vi "Get Config.vi"(8 "error in (no error)":errorcluster, 11 "SimSyA in":refnum<class "SimSyA.lvclass">) -> (0 "error out":errorcluster, 1 "Config Data":variant, 3 "SimSyA out":refnum<class "SimSyA.lvclass">)   [LabVIEW 2014, in "SimSyA.lvlib" / "SimSyA.lvclass"]
uses:
  SimSyA.lvclass
  DriverMasterSync/build/DriverMasterSync.lvlibp/Modules/HAL/DriverMasterSync/DriverMasterSyncClass/DriverMasterSync.lvclass
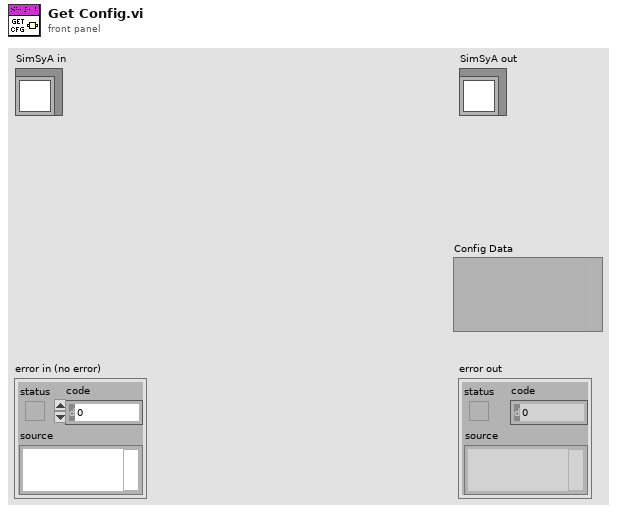
[diagram p1: front panel]
types:
  T1 = typedef "DriverMasterSync.lvlibp/HAL Config Data.ctl" = cluster{"HWSync Index":u32, "Driver Name":string, "Channel Mask":u64}
  T2 = cluster{"Channel Mask":u64, "SimSyA in":refnum<class "SimSyA.lvclass">}
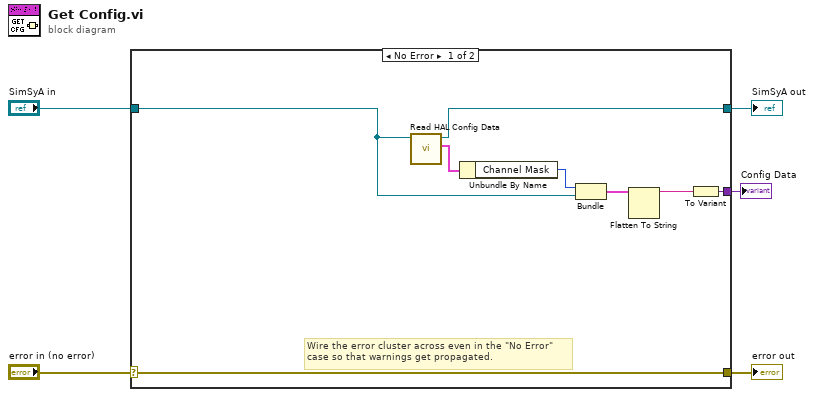
[diagram p0: block diagram]
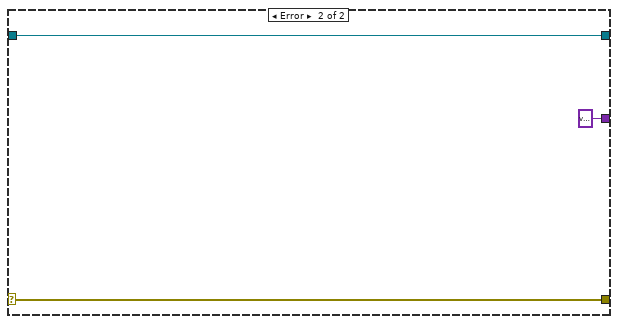
[diagram p2: hidden frame]
diagram:
  n1 = case shown="No Error" "error in (no error)" {
    selector: "error in (no error)" -> [w13 w16]
    tunnel: [w13 w16] -> w4
    tunnel: [w9 w15] -> w2
    tunnel: "SimSyA in" -> [w8 w15]
    tunnel: [w12 variant ("Variant")] -> w1
    frame No Error {
      # "Wire the error cluster across even in the \"No Error\"\ncase so that warnings get propagated."
      n2 = call "Read HAL Config Data.vi"("DriverMasterSync in"=w8) -> ("HAL Config Data"=w10:T1, "DriverMasterSync out"=w9:refnum<class "SimSyA.lvclass">)  [unwired: 8 in, 1 out]
      n3 = Unbundle By Name(w10) -> ("Channel Mask"=w11:u64)
      n4 = Bundle("Channel Mask"=w11, "SimSyA in"=w8) -> (w7:T2)  [unwired: 1 in]
      n5 = Flatten To String(anything=w7) -> (data string=w6:string)  [unwired: 3 in, 2 out]
      n6 = To Variant(anything=w6) -> (Variant=w12:variant)
    }
    frame Error {
    }
  }
  "error out" <- w4
  "SimSyA out" <- w2
  "Config Data" <- w1
